vi "Get Property from different hierarchy - Create Direction Subfolder.vi"(8 "error in":errorcluster, 11 "section ref":u64) -> (0 "error out":errorcluster, 3 "Value":bool)   [LabVIEW 2023, in "Ballard MIL-STD-1553 Scripting.lvlib"]
uses:
  Ballard MIL-STD-1553 Scripting.lvlib
  Constants.vi
  <vilib>/NI VeriStand/Custom Device API/Custom Device API.lvlib
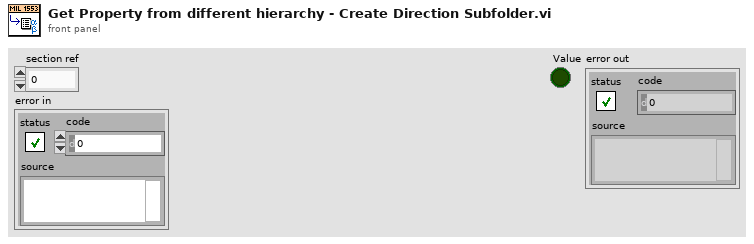
[diagram p1: front panel]
types:
  T1 = typedef "Custom Device API.lvlib/Custom Device Item Ref.ctl" = u64
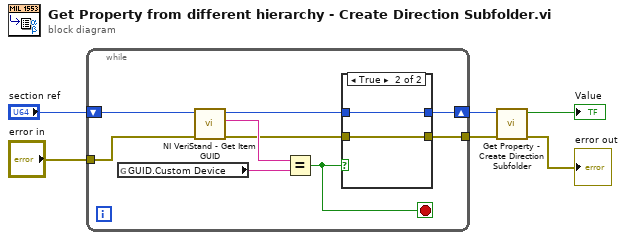
[diagram p0: block diagram]
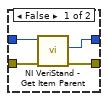
[diagram p2: hidden frame]
diagram:
  n1 = while {
    shift-right: [w15] -> w1
    shift-left: "section ref" -> [w13]
    tunnel: "error in" -> [w10]
    tunnel: [w14] -> w2
    stop <- w8 stop-if-true
    n2 = global read "Constants.vi" "GUID.Custom Device"() -> (w7:string)
    n3 = call <vilib>:"NI VeriStand - Get Item GUID.vi"("error in (no error)"=w10, "Item Ref in"=w13) -> ("error out"=w9:errorcluster, "GUID"=w11:string, "Item Ref out"=w12:T1)  [unwired: 7 in]
    n4 = Equal?(x=w11, y=w7) -> (x = y?=w8:bool)
    n5 = case shown="True" w8 {
      tunnel: w12 -> [w19 w21]
      tunnel: [w16 w21] -> w15
      tunnel: w9 -> [w17 w20]
      tunnel: [w18 w20] -> w14
      frame False {
        n6 = call <vilib>:"NI VeriStand - Get Item Parent.vi"("error in (no error)"=w17, "Item Ref in"=w19) -> ("error out"=w18:errorcluster, "Parent Ref"=w16:T1)  [unwired: 6 in, 2 out]
      }
      frame True {
      }
    }
  }
  n7 = call "Get Property - Create Direction Subfolder.vi"("error in"=w2, "custom device"=w1) -> ("error out"=→"error out":errorcluster, "Value"=→"Value":bool)  [unwired: 8 in]
